vi "Demo of fixed background.vi"() -> ()   [LabVIEW 2015]
uses:
  <vilib>/Platform/TimedLoop/XDataNode/timing_clust.ctl
  <vilib>/Platform/TimedLoop/XDataNode/nitl_modes.ctl
  <vilib>/Platform/TimedLoop/XDataNode/wakeup.ctl
  <vilib>/Platform/TimedLoop/XDataNode/XDataNode.xnode
  <vilib>/Platform/TimedLoop/XDataNode/XDNodeRunTimeDep.lvlib
panel:
  out "Array":dbl[](array[numeric])
  out "Iteration #":i32
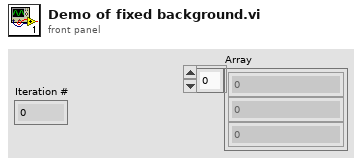
[diagram p1: front panel]
types:
  T1 = typedef "XDNodeRunTimeDep.lvlib/timing_clust.ctl" = cluster{"Expected End [f-1]":u64, "Actual End [f-1]":u64, "Finished Late? [f-1]":bool, "Expected End [i-1]":u64, "Actual End [i-1]":u64, "Finished Late? [i-1]":bool, "Expected Start [i]":u64, "Actual Start [i]":u64, "Expected Start [f]":u64, "Actual Start [f]":u64, "Source Name":string, "Structure Name":string, "Period":i64, "Deadline":i64, "Offset":i64, "Start":i64, "Priority":i32, "Timeout":i32, "Mode":T2, "Wakeup Reason":T3, "Error":errorcluster, "Source Type":string, "Secondary Source Type":string, "Global End Time":u64, "Global Start Time":u64, "Frame Duration":u64, "Iteration Duration":u64, "Assigned CPU":i32, "I/O Scan Engine Mode":u32}
  T2 = typedef "XDNodeRunTimeDep.lvlib/nitl_modes.ctl" = enum32{"No Change", "Process missed periods, maintain original phase", "Discard missed periods, maintain original phase", "Process missed periods, ignore original phase", "Discard missed periods, ignore original phase"}
  T3 = typedef "XDNodeRunTimeDep.lvlib/wakeup.ctl" = enum32{"Normal", "Aborted", "Asynchronous wakeup", "Timing source error", "Timed loop error", "Timeout"}
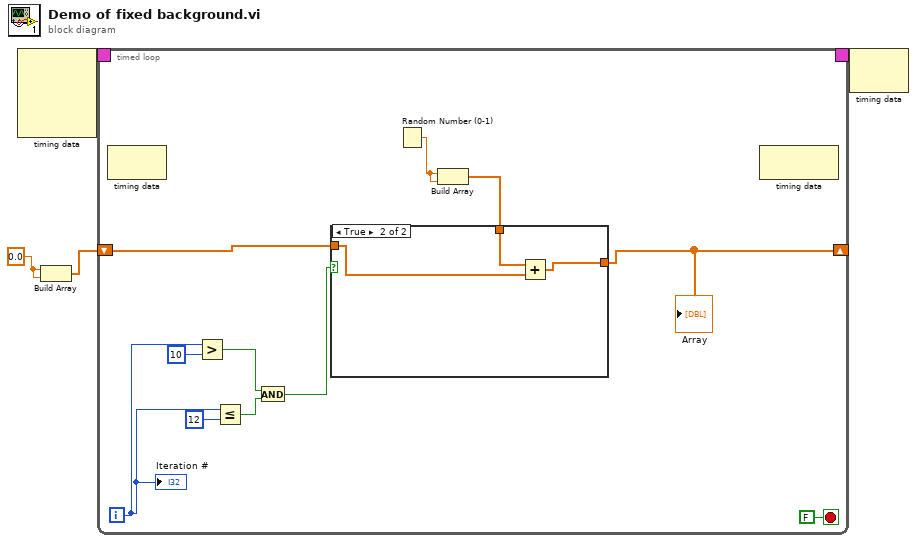
[diagram p0: block diagram]
diagram:
  w2 = 0.0 ("number: 0 to 1")
  n1 = node-c288() -> (w4:T1)  [unwired: 4 in]
  n2 = Build Array(w2, w2) -> (w1:dbl[])
  n3 = timed-loop {
    timing: w4 -> [_]
    timing-out: [_] -> w3
    shift-right: [w6] -> _
    shift-left: w1 -> [w5]
    i -> [w14]
    stop <- FALSE stop-if-true
    n4 = node-c288() -> ()  [unwired: 1 in, 1 out]
    n5 = Greater?(x=w14, y=10) -> (0:w11:bool)
    n6 = Less Or Equal?(x=w14, y=12) -> (x <= y?=w10:bool)
    n7 = And(x=w11, y=w10) -> (x .and. y?=w9:bool)
    n8 = Random Number (0-1)() -> (number: 0 to 1=w8:dbl)
    n9 = Build Array(w8, w8) -> (w7:dbl[])
    n10 = case shown="True" w9 {
      tunnel: [w16 w17] -> w6
      tunnel: w7 -> [_ w19]
      tunnel: w5 -> [w16 w18]
      frame False {
      }
      frame True {
        n11 = Add(x=w19, y=w18) -> (x+y=w17:dbl[])
      }
    }
    "Array" <- w6
    n12 = node-c288() -> ()  [unwired: 1 in, 1 out]
    "Iteration #" <- w14
  }
  n13 = node-c288(w3) -> ()  [unwired: 1 out]
